vi "open_shooter.vi"(8 "error in (no error)":errorcluster) -> (0 "error out":errorcluster)   [LabVIEW 2020]
uses:
  Status Frame Stuff/Talon Status Config Array.ctl
  Status Frame Stuff/Talon Status Frame Setting.ctl
  <vilib>/Rock Robotics/WPI/ThirdParty/Phoenix-LabVIEW/Motor Controller/Controls/CTRE_Phoenix_MotorControl_StatusFrameEnhanced.ctl
  Status Frame Stuff/STATUS_Period.ctl
  <vilib>/Rock Robotics/WPI/ThirdParty/Phoenix-LabVIEW/Motor Controller/Controls/CTRE_Phoenix_MotorControl_NeutralMode.ctl
  <vilib>/Rock Robotics/WPI/ThirdParty/REV Robotics/REVLib/Typedef/Spark MAX Idle Mode.ctl
panel:
  in  "Flywheel PIDF Constants":T1={"Set Constants"=TRUE, "P"=0.1, "I"=0.001, "D"=0.0, "F"=0.0461, "I Zone"=1000.0, "Cruise Velocity"=0, "Acceleration"=0, "Percent Deadband"=0.0}
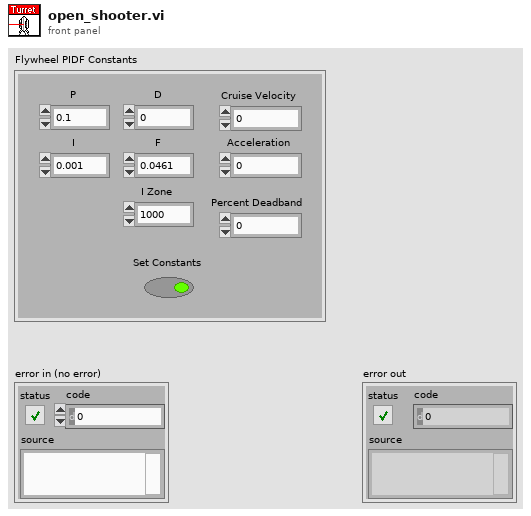
[diagram p1: front panel]
types:
  T1 = cluster{"Set Constants":bool, "P":dbl, "I":dbl, "D":dbl, "F":dbl, "I Zone":dbl, "Cruise Velocity":i32, "Acceleration":i32, "Percent Deadband":dbl}
  T2 = typedef "CTRE_Phoenix_MotorControl_NeutralMode.ctl" = enum8{"EEPROMSetting", "Override to Coast", "Override to Brake"}
  T3 = typedef "Talon Status Config Array.ctl" = T4[]
  T4 = typedef "Talon Status Frame Setting.ctl" = cluster{"Status Frame Enum":T5, "STATUS_Period":T6}
  T5 = typedef "CTRE_Phoenix_MotorControl_StatusFrameEnhanced.ctl" = u16
  T6 = typedef "STATUS_Period.ctl" = i32
  T7 = typedef "WPI_MotorControlDeviceRef.ctl" = cluster{"DeviceStatus":errorcluster, "Type":T8, "PWM":cluster{"PWM Channel":T9, "DeadBand":T10}, "CAN":cluster{"Device Number":u8, "SetOutput VI Ref":variant, "GetOutput VI Ref":variant, "Enable VI Ref":variant, "Disable VI Ref":variant, "Data":variant}, "Invert":bool, "DIO PWM":cluster{"PWM \"Enable\" Channel":T9, "DIOChannel":T11, "PWM Rate":dbl}}
  T8 = typedef "WPI_MotorControlType.ctl" = enum16{"PWM", "CAN", "DIO PWM"}
  T9 = typedef "FPGA_DIOPWMChannel.ctl" = enum8{"PWM 0", "PWM 1", "PWM 2", "PWM 3", "PWM 4", "PWM 5", "PWM 6", "PWM 7", "PWM 8", "PWM 9", "PWM MXP 0", "PWM MXP 1", "PWM MXP 2", "PWM MXP 3", "PWM MXP 4", "PWM MXP 5", "PWM MXP 6", "PWM MXP 7", "PWM MXP 8", "PWM MXP 9", "Invalid"}
  T10 = typedef "WPI_PWMDeadband.ctl" = cluster{"Name":string, "maxPositivePwm":i32, "minPositivePwm":i32, "centerPwm":i32, "maxNegativePwm":i32, "minNegativePwm":i32, "angularRange":u16}
  T11 = typedef "FPGA_DIOChannel.ctl" = enum8{"DIO 0", "DIO 1", "DIO 2", "DIO 3", "DIO 4", "DIO 5", "DIO 6", "DIO 7", "DIO 8", "DIO 9", "DIO MXP 0", "DIO MXP 1", "DIO MXP 2", "DIO MXP 3", "DIO MXP 4", "DIO MXP 5", "DIO MXP 6", "DIO MXP 7", "DIO MXP 8", "DIO MXP 9", "DIO MXP 10", "DIO MXP 11", "DIO MXP 12", "DIO MXP 13", "DIO MXP 14", "DIO MXP 15", "SPI Port CS1", "SPI Port CS2", "SPI Port CS3", "SPI Port MISO", "SPI Port MOSI", "Invalid"}
  T12 = typedef "Spark MAX Idle Mode.ctl" = enum16{"Coast", "Brake"}
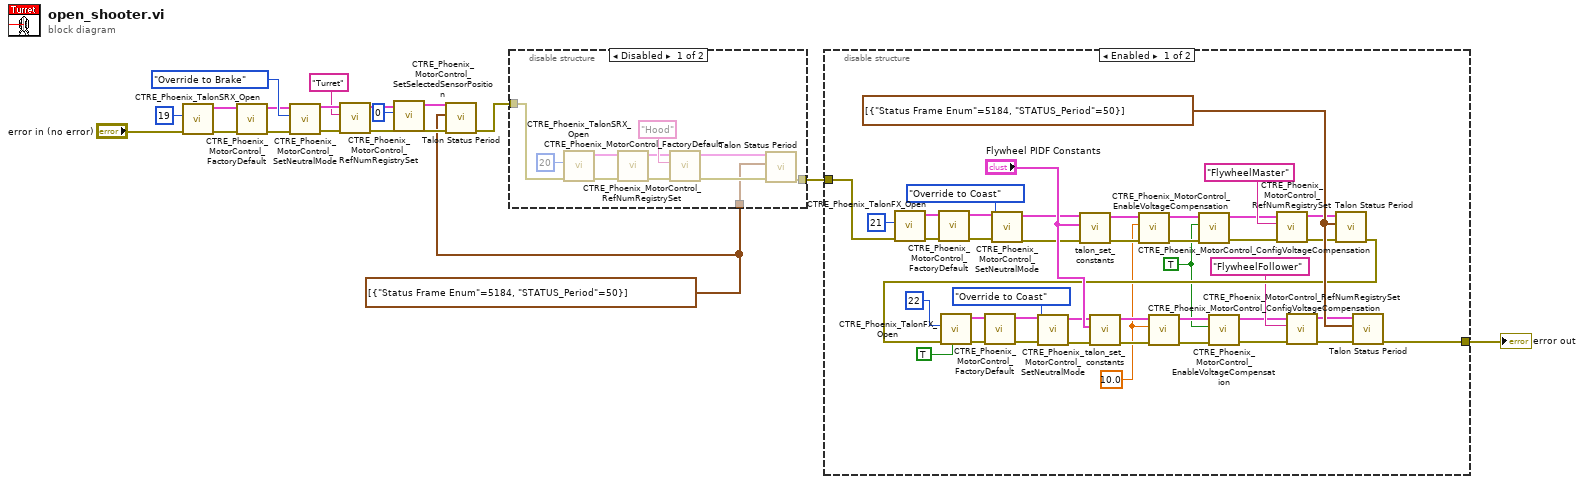
[diagram p0: block diagram]
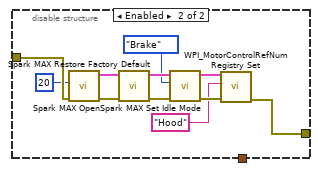
[diagram p3: hidden frame]
diagram:
  w2 = T3 [{"Status Frame Enum"=5184, "STATUS_Period"=50}] ("Drive Status Config")
  n1 = call <vilib>:"CTRE_Phoenix_TalonSRX_Open.vi"("error in"="error in (no error)", "Device Number"=u8 19) -> ("error out"=w8:errorcluster, "PhoenixMotorControlDevRef"=w9:T7)  [unwired: 8 in]
  n2 = call <vilib>:"CTRE_Phoenix_MotorControl_FactoryDefault.vi"("error in"=w8, "PhoenixMotorControlDevRef"=w9) -> ("error out"=w18:errorcluster, "PhoenixMotorControlDevRef"=w15:T7)  [unwired: 8 in]
  n3 = call <vilib>:"CTRE_Phoenix_MotorControl_SetNeutralMode.vi"("error in (no error)"=w18, "Motor Control Neutral Mode"=CTRE_Phoenix_MotorControl_NeutralMode."Override to Brake", "PhoenixMotorControlDevRef"=w15) -> ("error out"=w17:errorcluster, "PhoenixMotorControlDevRef"=w16:T7)  [unwired: 7 in]
  n4 = call <vilib>:"CTRE_Phoenix_MotorControl_RefNumRegistrySet.vi"("error in (no error)"=w17, "refnum name"="Turret", "PhoenixMotorControlDevRef"=w16) -> ("error out"=w7:errorcluster, "PhoenixMotorControlDevRef"=w6:T7)  [unwired: 7 in]
  n5 = call <vilib>:"CTRE_Phoenix_MotorControl_SetSelectedSensorPosition.vi"("error in (no error)"=w7, "New Sensor Position"=0, "PhoenixMotorControlDevRef"=w6) -> ("error out"=w4:errorcluster, "PhoenixMotorControlDevRef"=w5:T7)  [unwired: 7 in]
  n6 = call "Talon Status Period.vi"("error in (no error)"=w4, "Status Config Array"=w2, "PhoenixMotorControlDevRef"=w5) -> ("error out"=w13:errorcluster)  [unwired: 7 in, 1 out]
  n7 = disable-structure shown="Disabled" {
    disable-tunnel: [w30 w31] -> w14
    disable-tunnel: w13 -> [w27 w41]
    disable-tunnel: w2 -> [w20 _]
    frame Disabled {
      n8 = call <vilib>:"CTRE_Phoenix_TalonSRX_Open.vi"("error in"=w27, "Device Number"=u8 20) -> ("error out"=w21:errorcluster, "PhoenixMotorControlDevRef"=w22:T7)  [unwired: 8 in]
      n9 = call <vilib>:"CTRE_Phoenix_MotorControl_FactoryDefault.vi"("error in"=w21, "PhoenixMotorControlDevRef"=w22) -> ("error out"=w23:errorcluster, "PhoenixMotorControlDevRef"=w24:T7)  [unwired: 8 in]
      n10 = call <vilib>:"CTRE_Phoenix_MotorControl_RefNumRegistrySet.vi"("error in (no error)"=w23, "refnum name"="Hood", "PhoenixMotorControlDevRef"=w24) -> ("error out"=w29:errorcluster, "PhoenixMotorControlDevRef"=w28:T7)  [unwired: 7 in]
      n11 = call "Talon Status Period.vi"("error in (no error)"=w29, "Status Config Array"=w20, "PhoenixMotorControlDevRef"=w28) -> ("error out"=w30:errorcluster)  [unwired: 7 in, 1 out]
    }
    frame Enabled {
      n12 = call <vilib>:"Spark MAX Open.vi"("error in (no error)"=w41, "Device Number"=u8 20) -> ("error out"=w38:errorcluster, "MotorControlDeviceRef"=w39:T7)  [unwired: 8 in]
      n13 = call <vilib>:"Spark MAX Restore Factory Default.vi"("error in"=w38, "MotorControlDeviceRef"=w39) -> ("error out"=w37:errorcluster, "MotorControlDeviceRef"=w36:T7)  [unwired: 8 in]
      n14 = call <vilib>:"Spark MAX Set Idle Mode.vi"("error in (no error)"=w37, "Idle Mode"=Spark_MAX_Idle_Mode."Brake", "MotorControlDeviceRef in"=w36) -> ("error out"=w34:errorcluster, "MotorControlDeviceRef out"=w33:T7)  [unwired: 7 in]
      n15 = call <vilib>:"WPI_MotorControlRefNum Registry Set.vi"("error in (no error)"=w34, "refnum name"="Hood", "MotorControlDevRef"=w33) -> ("error out"=w31:errorcluster)  [unwired: 7 in, 1 out]
    }
  }
  n16 = disable-structure shown="Enabled" {
    disable-tunnel: w14 -> [w57 w84]
    disable-tunnel: [w56 w84] -> w1
    frame Enabled {
      w46 = TRUE ("Enable Voltage Compensation?")
      w47 = 10.0 ("Saturation Voltage")
      w78 = T3 [{"Status Frame Enum"=5184, "STATUS_Period"=50}] ("Drive Status Config")
      n17 = call <vilib>:"CTRE_Phoenix_TalonFX_Open.vi"("error in"=w57, "Device Number"=u8 21) -> ("error out"=w58:errorcluster, "PhoenixMotorControlDevRef"=w59:T7)  [unwired: 8 in]
      n18 = call <vilib>:"CTRE_Phoenix_MotorControl_FactoryDefault.vi"("error in"=w58, "PhoenixMotorControlDevRef"=w59) -> ("error out"=w63:errorcluster, "PhoenixMotorControlDevRef"=w62:T7)  [unwired: 8 in]
      n19 = call <vilib>:"CTRE_Phoenix_MotorControl_SetNeutralMode.vi"("error in (no error)"=w63, "Motor Control Neutral Mode"=CTRE_Phoenix_MotorControl_NeutralMode."Override to Coast", "PhoenixMotorControlDevRef"=w62) -> ("error out"=w80:errorcluster, "PhoenixMotorControlDevRef"=w79:T7)  [unwired: 7 in]
      n20 = call "talon_set_constants.vi"("error in"=w80, "Constants"="Flywheel PIDF Constants", "PhoenixMotorControlDevRef"=w79) -> ("error out"=w55:errorcluster, "PhoenixMotorControlDevRef"=w54:T7)  [unwired: 7 in]
      n21 = call <vilib>:"CTRE_Phoenix_MotorControl_ConfigVoltageCompensation.vi"("error in (no error)"=w55, "Saturation Voltage"=w47, "PhoenixMotorControlDevRef"=w54) -> ("error out"=w53:errorcluster, "PhoenixMotorControlDevRef"=w52:T7)  [unwired: 7 in]
      n22 = call <vilib>:"CTRE_Phoenix_MotorControl_EnableVoltageCompensation.vi"("error in (no error)"=w53, "Enable Voltage Compensation?"=w46, "PhoenixMotorControlDevRef"=w52) -> ("error out"=w44:errorcluster, "PhoenixMotorControlDevRef"=w45:T7)  [unwired: 7 in]
      n23 = call <vilib>:"CTRE_Phoenix_MotorControl_RefNumRegistrySet.vi"("error in (no error)"=w44, "refnum name"="FlywheelMaster", "PhoenixMotorControlDevRef"=w45) -> ("error out"=w75:errorcluster, "PhoenixMotorControlDevRef"=w77:T7)  [unwired: 7 in]
      n24 = call "Talon Status Period.vi"("error in (no error)"=w75, "Status Config Array"=w78, "PhoenixMotorControlDevRef"=w77) -> ("error out"=w76:errorcluster)  [unwired: 7 in, 1 out]
      n25 = call <vilib>:"CTRE_Phoenix_TalonFX_Open.vi"("Invert"=TRUE, "error in"=w76, "Device Number"=u8 22) -> ("error out"=w65:errorcluster, "PhoenixMotorControlDevRef"=w66:T7)  [unwired: 7 in]
      n26 = call <vilib>:"CTRE_Phoenix_MotorControl_FactoryDefault.vi"("error in"=w65, "PhoenixMotorControlDevRef"=w66) -> ("error out"=w70:errorcluster, "PhoenixMotorControlDevRef"=w69:T7)  [unwired: 8 in]
      n27 = call <vilib>:"CTRE_Phoenix_MotorControl_SetNeutralMode.vi"("error in (no error)"=w70, "Motor Control Neutral Mode"=CTRE_Phoenix_MotorControl_NeutralMode."Override to Coast", "PhoenixMotorControlDevRef"=w69) -> ("error out"=w82:errorcluster, "PhoenixMotorControlDevRef"=w81:T7)  [unwired: 7 in]
      n28 = call "talon_set_constants.vi"("error in"=w82, "Constants"="Flywheel PIDF Constants", "PhoenixMotorControlDevRef"=w81) -> ("error out"=w49:errorcluster, "PhoenixMotorControlDevRef"=w48:T7)  [unwired: 7 in]
      n29 = call <vilib>:"CTRE_Phoenix_MotorControl_ConfigVoltageCompensation.vi"("error in (no error)"=w49, "Saturation Voltage"=w47, "PhoenixMotorControlDevRef"=w48) -> ("error out"=w50:errorcluster, "PhoenixMotorControlDevRef"=w51:T7)  [unwired: 7 in]
      n30 = call <vilib>:"CTRE_Phoenix_MotorControl_EnableVoltageCompensation.vi"("error in (no error)"=w50, "Enable Voltage Compensation?"=w46, "PhoenixMotorControlDevRef"=w51) -> ("error out"=w42:errorcluster, "PhoenixMotorControlDevRef"=w43:T7)  [unwired: 7 in]
      n31 = call <vilib>:"CTRE_Phoenix_MotorControl_RefNumRegistrySet.vi"("error in (no error)"=w42, "refnum name"="FlywheelFollower", "PhoenixMotorControlDevRef"=w43) -> ("error out"=w74:errorcluster, "PhoenixMotorControlDevRef"=w73:T7)  [unwired: 7 in]
      n32 = call "Talon Status Period.vi"("error in (no error)"=w74, "Status Config Array"=w78, "PhoenixMotorControlDevRef"=w73) -> ("error out"=w56:errorcluster)  [unwired: 7 in, 1 out]
    }
    frame Disabled {
    }
  }
  "error out" <- w1
